vi "Main.vi"() -> ()   [LabVIEW 2016]
uses:
  type defs/action buttons.ctl
  type defs/mode buttons.ctl
  <vilib>/picture/picture.llb/imagedata.ctl
  type defs/state.ctl
  type defs/data.ctl
  <vilib>/vision/Image Controls.llb/IMAQ Image.ctl
  type defs/task.ctl
  <vilib>/vision/NI_Vision_Development_Module.lvlib
panel:
  in  "# máximo\nde iterações":i32
  out "image":u8[](array[numeric])
  out "image data":T1
  out "Array":T2(array[cluster])
  in  "K":u16
  in  "threshold (0 a 255)":u8
  out "Frame Rate":dbl
  in  "mode buttons":T3
  out "image display":T4(plugin-control)
  in  "action buttons":T5
  in  "Stop":bool
  # "Machine\nVision\nApp"
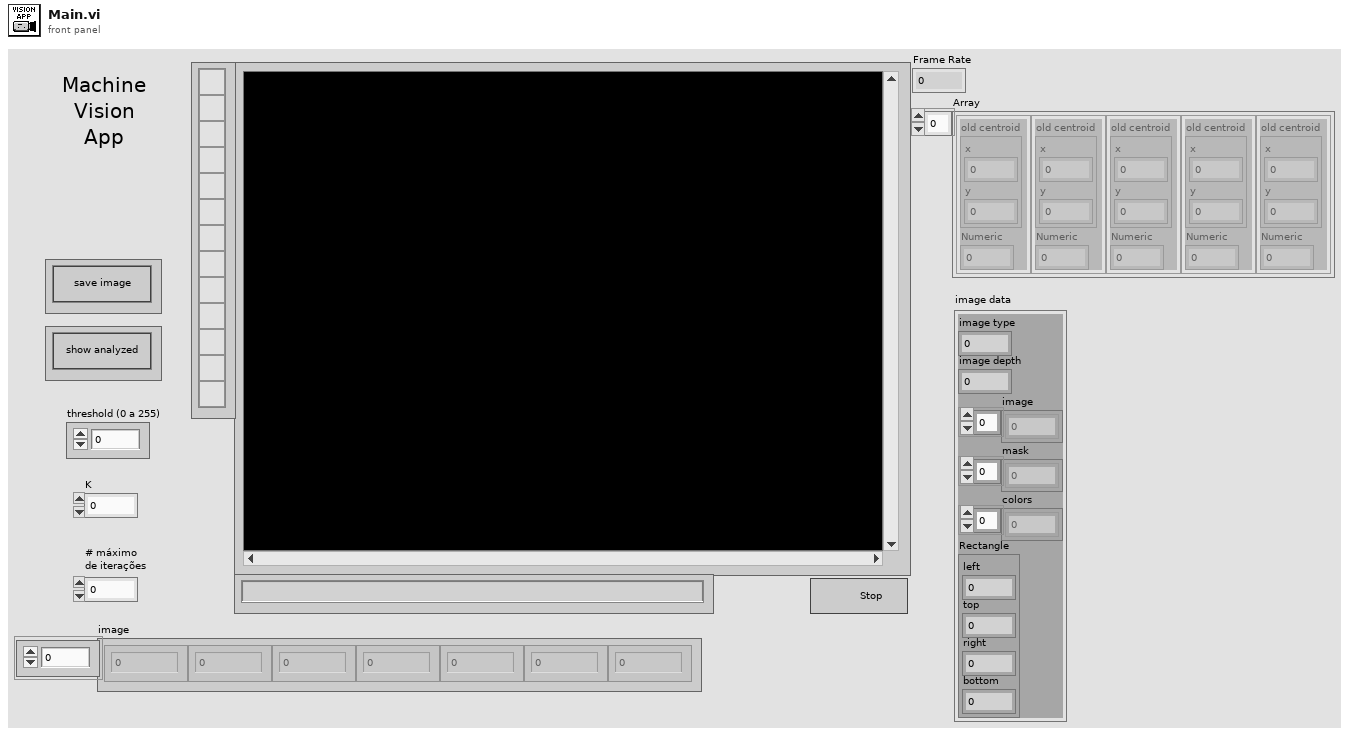
[diagram p1: front panel]
types:
  T1 = typedef "imagedata.ctl" = cluster{"image type":i32, "image depth":i32, "image":u8[], "mask":u8[], "colors":u32[], "Rectangle":cluster{"left":i16, "top":i16, "right":i16, "bottom":i16}}
  T2 = cluster{"old centroid":cluster{"x":dbl, "y":dbl}, "Numeric":i32}[]
  T3 = typedef "mode buttons.ctl" = cluster{"show analyzed":bool}
  T4 = typedef "IMAQ Image.ctl" = refnum<image>
  T5 = typedef "action buttons.ctl" = cluster{"save image":bool}
  T6 = typedef "data.ctl" = cluster{"save image":bool, "qsm":cluster{"Webcam image ref":T4, "Analyzed image ref":T4, "Stop webcam":bool}}
  T7 = typedef "state.ctl" = enum16{"(qsm) schedule", "(qsm) initialize", "(qsm) release", "(qsm) clean up", "(qsm) shutdown", "(myRIO) initialize", "(myRIO) clean up", "(myRIO) update ports", "(image) get", "(image) analyze", "(image) overlay", "(image) show", "save image", "state A", "state B", "state C", "state D", "state E", "state F", "state G", "state H"}
  T8 = cluster{"Desired Font (Application)":enum16{"User-specified Font", "Application Font", "System Font", "Dialog Font"}, "[User-specified Font]":cluster{"Font Name":string, "Size":i16, "Strikeout?":bool, "Italic?":bool, "Underline?":bool, "Outline?":bool, "Shadow?":bool, "Bold?":bool, "Rotation Angle":dbl}, "Horizontal Alignment":i16, "Vertical Alignment":i16}
  T9 = typedef "task.ctl" = T7[]
  T10 = typedef "Image Type" = u32
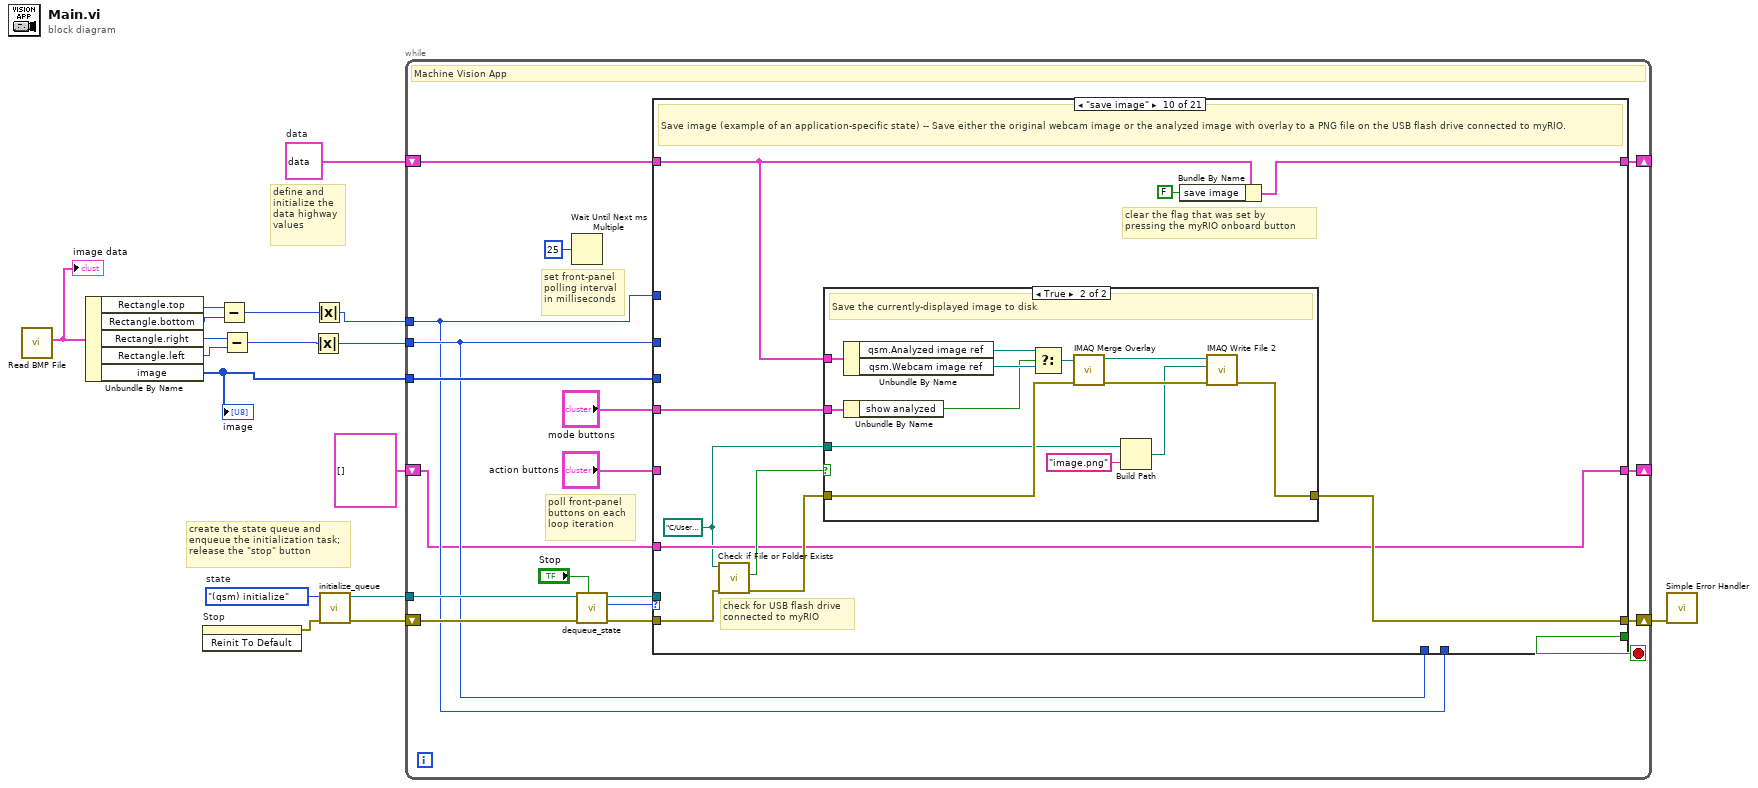
[diagram p0: block diagram]
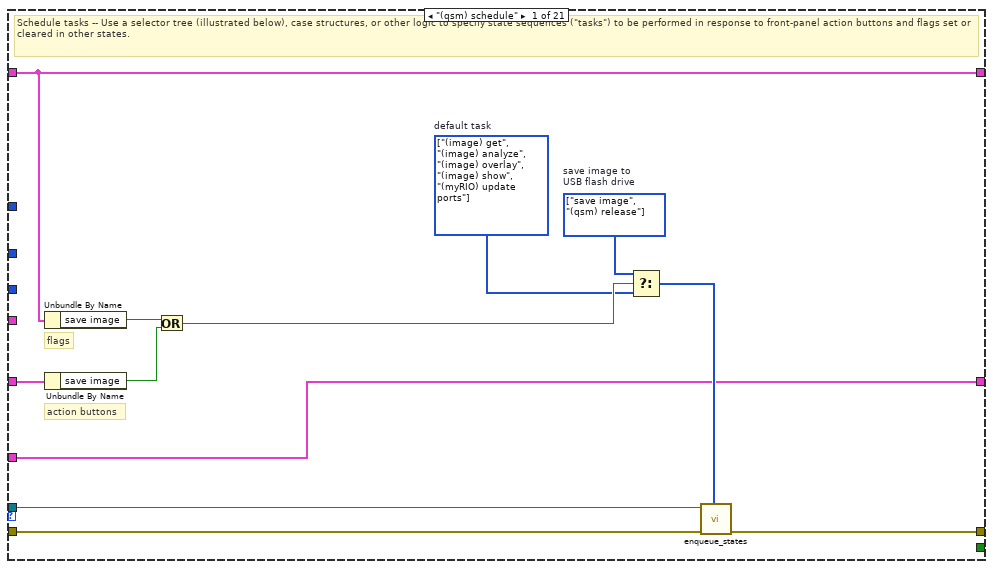
[diagram p2: hidden frame]
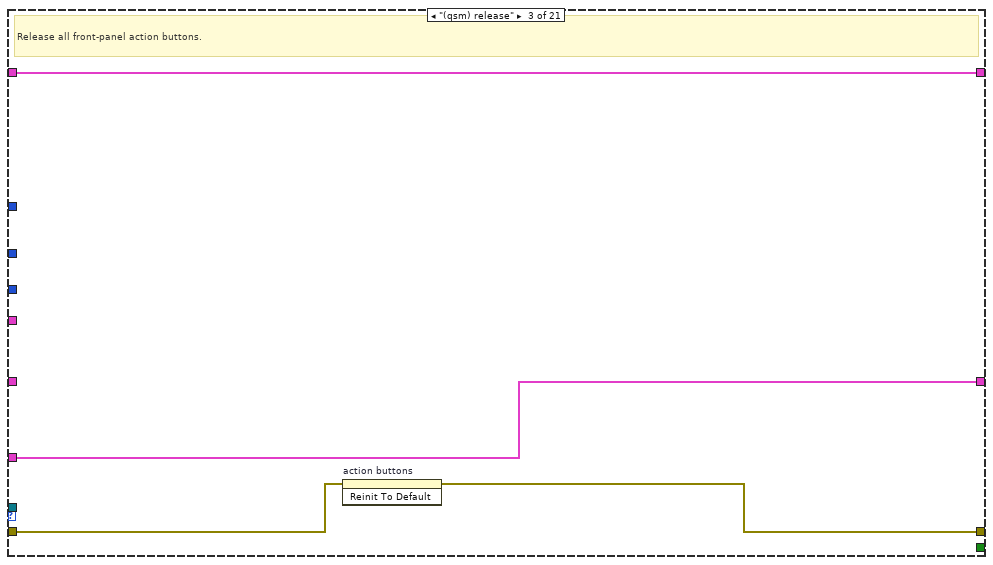
[diagram p4: hidden frame]
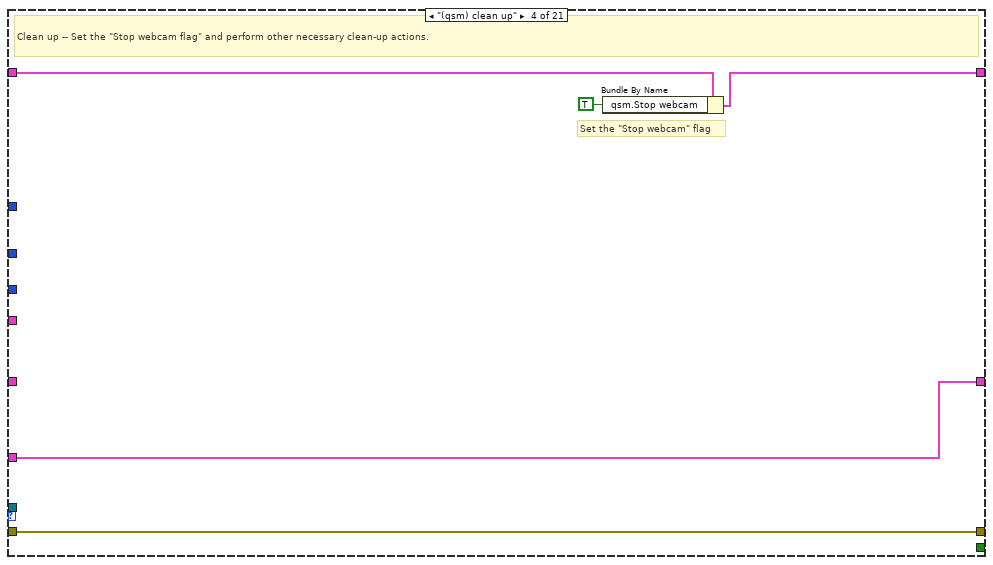
[diagram p5: hidden frame]
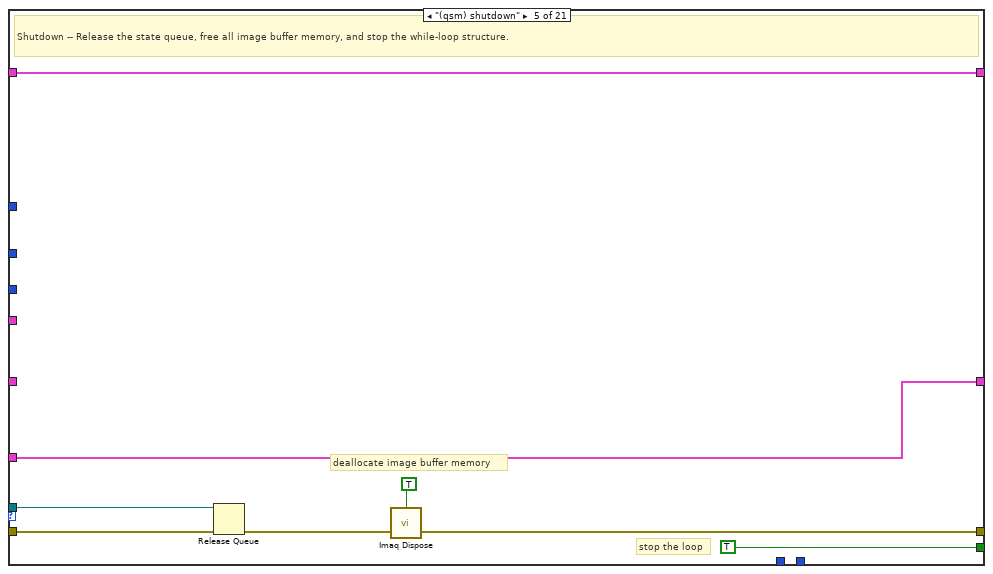
[diagram p6: hidden frame]
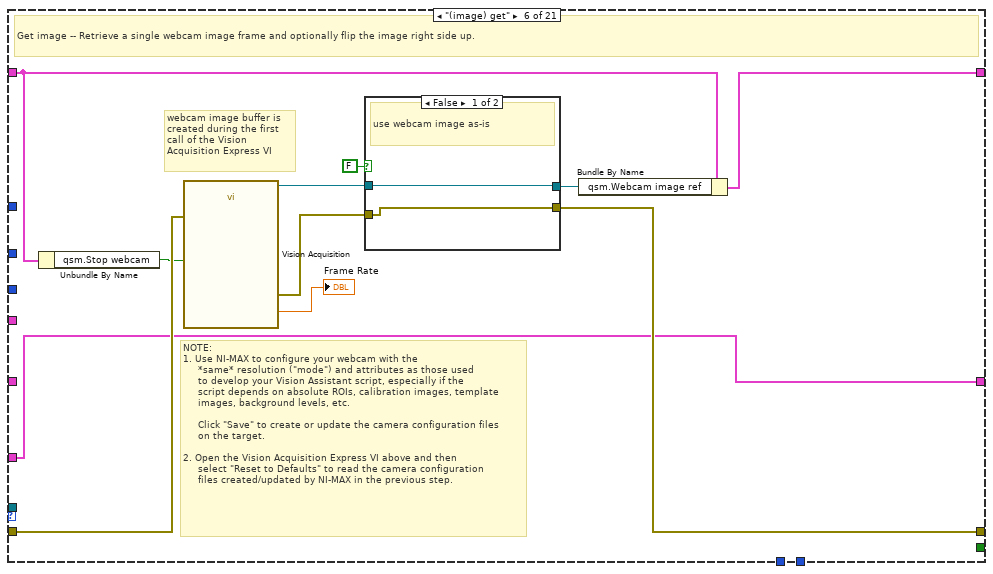
[diagram p7: hidden frame]
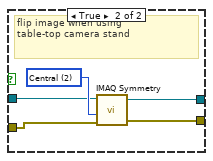
[diagram p8: hidden frame]
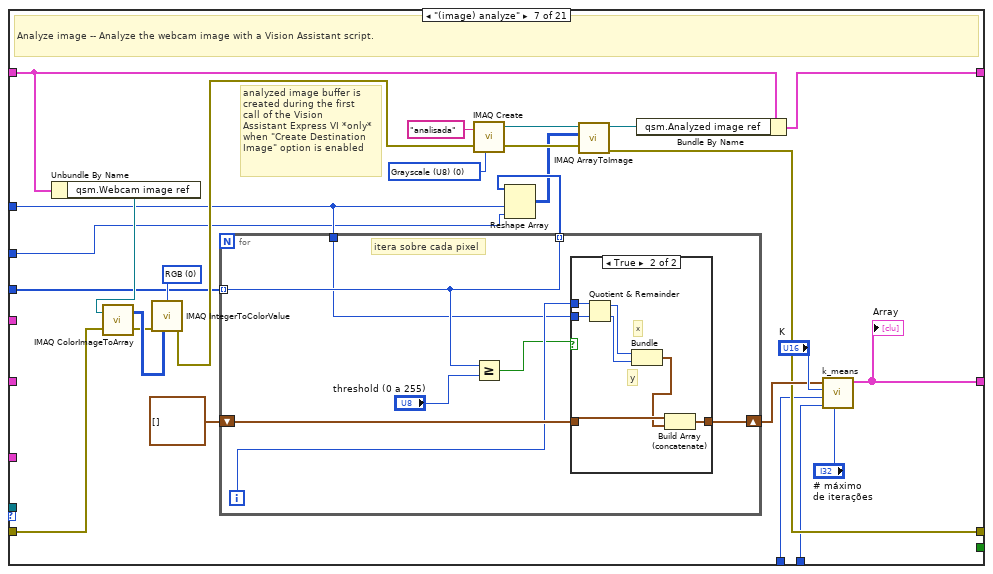
[diagram p9: hidden frame]
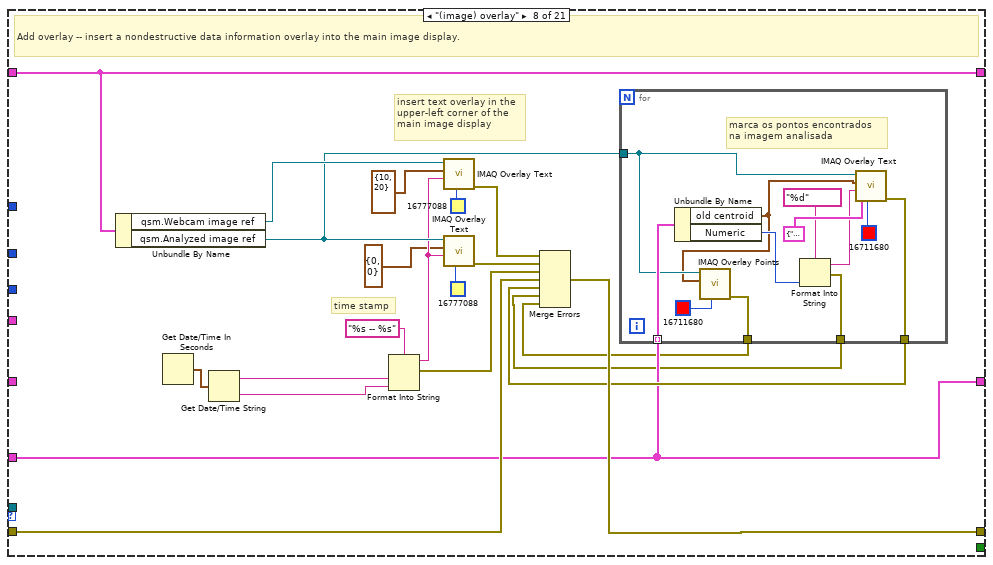
[diagram p11: hidden frame]
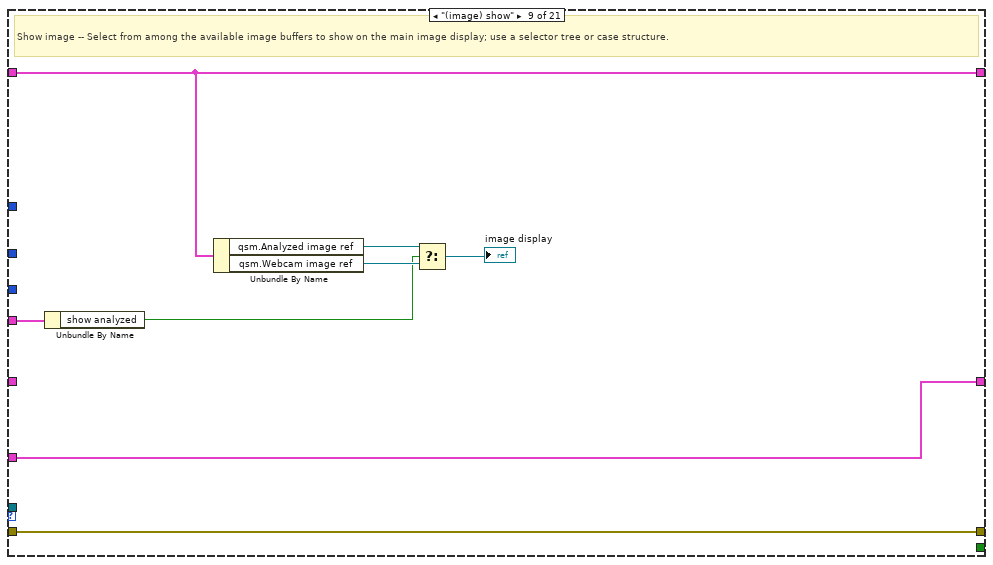
[diagram p12: hidden frame]
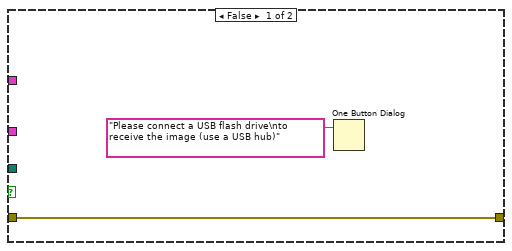
[diagram p13: hidden frame]
diagram:
  w16 = T6 {"save image"=FALSE, "qsm"={"Webcam image ref"=refnum, "Analyzed image ref"=refnum, "Stop webcam"=FALSE}}  # data
  w12 = state."(qsm) initialize"  # state
  # "define and \ninitialize the \ndata highway\nvalues"
  # "create the state queue and\nenqueue the initialization task;\nrelease the \"stop\" button"
  n1 = call <vilib>:"Read BMP File.vi"() -> ("image data"=w11:T1)  [unwired: 9 in, 2 out]
  "image data" <- w11
  n2 = Unbundle By Name(w11) -> ("Rectangle.top"=w7:i16, "Rectangle.bottom"=w6:i16, "Rectangle.right"=w9:i16, "Rectangle.left"=w8:i16, "image"=w10:u8[])
  "image" <- w10
  n3 = invoke on="Stop" class="Bool" method="Reinit To Default"() -> (error out=w13:errorcluster)  [unwired: 3 in, 2 out]
  n4 = Subtract(x=w7, y=w6) -> (x-y=w5:i16)
  n5 = Subtract(x=w9, y=w8) -> (x-y=w3:i16)
  n6 = Absolute Value(x=w3) -> (abs(x)=w2:i16)
  n7 = Absolute Value(x=w5) -> (abs(x)=w4:i16)
  n8 = call "initialize_queue.vi"("error in (no error)"=w13, "state"=w12) -> ("error out"=w15:errorcluster, "queue out"=w14:refnum<queue>)  [unwired: 8 in]
  n9 = while {
    shift-right: [w23] -> w17
    shift-left: w15 -> [w31]
    tunnel: w14 -> [w32]
    shift-right: [w25] -> _
    shift-left: w16 -> [w34]
    tunnel: w10 -> [w22]
    tunnel: w4 -> [w20]
    tunnel: w2 -> [w21]
    shift-right: [w19] -> _
    shift-left: T2 [] ("Array") -> [w18]
    stop <- w33 stop-if-true
    # "set front-panel\npolling interval\nin milliseconds"
    # "poll front-panel\nbuttons on each\nloop iteration"
    # "Machine Vision App"
    n10 = Wait Until Next ms Multiple(millisecond multiple=u32 25) -> ()  [unwired: 1 out]
    n11 = call "dequeue_state.vi"("stop"="Stop", "error in (no error)"=w31, "queue in"=w32) -> ("error out"=w24:errorcluster, "state"=w26:T7, "queue out"=w29:refnum<queue>)  [unwired: 6 in]
    n12 = case shown="\"save image\"" w26 {
      tunnel: w29 -> [w45 _ _ _ w65 _ _ _ _ _ _ _ _ _ _ _ _ _ _ _ _]
      tunnel: "action buttons" -> [w47 _ _ _ _ _ _ _ _ _ _ _ _ _ _ _ _ _ _ _ _]
      tunnel: w34 -> [w46 w50 w54 w58 w64 w72 w111 w136 w164 w177 w195 w198 w201 w204 w207 w210 w213 w216 w219 w222 w225]
      tunnel: [_ _ _ _ TRUE _ _ _ _ _ _ _ _ _ _ _ _ _ _ _ _] -> w33
      tunnel: "mode buttons" -> [_ _ _ _ _ _ _ _ w163 w173 _ _ _ _ _ _ _ _ _ _ _]
      tunnel: [w46 w50 w54 w57 w64 w77 w110 w136 w164 w176 w195 w198 w201 w204 w207 w210 w213 w216 w219 w222 w225] -> w25
      tunnel: w24 -> [w44 w49 w53 w56 w66 w78 w97 w135 w161 w174 w194 w197 w200 w203 w206 w209 w212 w215 w218 w221 w224]
      tunnel: [w37 w49 w52 w56 w61 w70 w96 w134 w161 w170 w194 w197 w200 w203 w206 w209 w212 w215 w218 w221 w224] -> w23
      tunnel: w22 -> [_ _ _ _ _ _ w95 _ _ _ _ _ _ _ _ _ _ _ _ _ _]
      tunnel: w20 -> [_ _ _ _ _ _ w90 _ _ _ _ _ _ _ _ _ _ _ _ _ _]
      tunnel: w21 -> [_ _ _ _ _ _ w89 _ _ _ _ _ _ _ _ _ _ _ _ _ _]
      tunnel: w21 -> [_ _ _ _ _ _ w88 _ _ _ _ _ _ _ _ _ _ _ _ _ _]
      tunnel: w20 -> [_ _ _ _ _ _ w87 _ _ _ _ _ _ _ _ _ _ _ _ _ _]
      tunnel: [w36 w48 w51 w55 w60 w68 w86 w131 w160 w169 w193 w196 w199 w202 w205 w208 w211 w214 w217 w220 w223] -> w19
      tunnel: w18 -> [w36 w48 w51 w55 w60 w68 _ w131 w160 w169 w193 w196 w199 w202 w205 w208 w211 w214 w217 w220 w223]
      frame "(qsm) schedule" {
        w40 = T9 [enum."save image", enum."(qsm) release"] items=["(qsm) schedule", "(qsm) initialize", "(qsm) release", "(qsm) clean up", "(qsm) shutdown", "(myRIO) initialize", "(myRIO) clean up", "(myRIO) update ports", "(image) get", "(image) analyze", "(image) overlay", "(image) show", "save image", "state A", "state B", "state C", "state D", "state E", "state F", "state G", "state H"]  # save image to USB flash drive
        w38 = T9 [enum."(image) get", enum."(image) analyze", enum."(image) overlay", enum."(image) show", enum."(myRIO) update ports"] items=["(qsm) schedule", "(qsm) initialize", "(qsm) release", "(qsm) clean up", "(qsm) shutdown", "(myRIO) initialize", "(myRIO) clean up", "(myRIO) update ports", "(image) get", "(image) analyze", "(image) overlay", "(image) show", "save image", "state A", "state B", "state C", "state D", "state E", "state F", "state G", "state H"]  # default task
        # "action buttons"
        # "flags"
        # "Schedule tasks -- Use a selector tree (illustrated below), case structures, or other logic to specify state sequences (\"tasks\") to be performed in response to front-panel action buttons and flags set or cleared in other states."
        n13 = Unbundle By Name "Unbundle By Name"(w46) -> ("save image"=w43:bool)
        n14 = Unbundle By Name(w47) -> ("save image"=w42:bool)
        n15 = Or(x=w43, y=w42) -> (x .or. y?=w41:bool)
        n16 = Select(t=w40, s=w41, f=w38) -> (s? t:f=w39:T9)
        n17 = call "enqueue_states.vi"("task"=w39, "error in"=w44, "queue in"=w45) -> ("error out"=w37:errorcluster)  [unwired: 7 in, 1 out]
      }
      frame "(qsm) initialize" {
        # "Initialize -- Allocate memory for additional image buffers, if necessary, and perform other one-time initialization steps."
      }
      frame "(qsm) release" {
        # "Release all front-panel action buttons."
        n18 = invoke on="action buttons" class="Clust (strict)" method="Reinit To Default"(error in=w53) -> (error out=w52:errorcluster)  [unwired: 2 in, 2 out]
      }
      frame "(qsm) clean up" {
        # "Set the \"Stop webcam\" flag"
        # "Clean up -- Set the \"Stop webcam flag\" and perform other necessary clean-up actions."
        n19 = Bundle By Name(cluster=w58, "qsm.Stop webcam"=TRUE) -> (w57:T6)
      }
      frame "(qsm) shutdown" {
        # "deallocate image buffer memory"
        # "stop the loop"
        # "Shutdown -- Release the state queue, free all image buffer memory, and stop the while-loop structure."
        n20 = Release Queue(queue=w65, error in (no error)=w66) -> (error out=w62:errorcluster)  [unwired: 1 in, 2 out]
        n21 = call "Imaq Dispose"("All Images? (No)"=TRUE, "error in (no error)"=w62) -> ("error out"=w61:errorcluster)  [unwired: 4 in]
      }
      frame "(image) get" {
        # "webcam image buffer is\ncreated during the first\ncall of the Vision\nAcquisition Express VI"
        # "NOTE:\n1. Use NI-MAX to configure your webcam with the\n     *same* resolution (\"mode\") and attributes as those used \n     to develop your Vision Assistant script, especially if the\n     script depends on absolute ROIs, calibration images, template\n     images, background levels, etc.\n \n     Click \"Save\" to create or update the camera configuration files\n     on the target.\n\n2. Open the Vision Acquisition Express VI above and then\n     select \"Reset to Defaults\" to read the camera configuration\n     files created/updated by NI-MAX in the previous step."
        # "Get image -- Retrieve a single webcam image frame and optionally flip the image right side up."
        n22 = Unbundle By Name(w72) -> ("qsm.Stop webcam"=w71:bool)
        n23 = call "Vision Acquisition"("Stop (F)"=w71, "error in"=w78) -> ("Image Out"=w76:T4, "Frame Rate"=→"Frame Rate":dbl, "error out"=w74:errorcluster)  [unwired: 22 in, 1 out]
        n24 = case shown="False" FALSE {
          tunnel: w76 -> [w80 w84]
          tunnel: [w80 w83] -> w75
          tunnel: w74 -> [w79 w82]
          tunnel: [w79 w81] -> w70
          frame False {
            # "use webcam image as-is"
          }
          frame True {
            w85 = u32 2 items=["Horizontal", "Vertical", "Central", "1st Diagonal", "2nd Diagonal"] ("Type of Symmetry")
            # "flip image when using\ntable-top camera stand"
            n25 = call "IMAQ Symmetry"("error in (no error)"=w82, "Type of Symmetry"=w85, "Image Src"=w84) -> ("error out"=w81:errorcluster, "Image Dst Out"=w83:T4)  [unwired: 2 in]
          }
        }
        n26 = Bundle By Name(cluster=w72, "qsm.Webcam image ref"=w75) -> (w77:T6)
      }
      frame "(image) analyze" {
        w105 = T10 0 items=["Grayscale (U8)", "Grayscale (I16)", "Grayscale (SGL)", "Complex (CSG)", "RGB (U32)", "HSL (U32)", "RGB (U64)", "Grayscale (U16)"] ("Image Type")
        w107 = u16 0 items=["RGB", "HSL", "HSV", "HSI"] ("Color Mode")
        # "analyzed image buffer is\ncreated during the first\ncall of the Vision\nAssistant Express VI *only*\nwhen \"Create Destination\nImage\" option is enabled"
        # "Analyze image -- Analyze the webcam image with a Vision Assistant script."
        n27 = Unbundle By Name "Unbundle By Name"(w111) -> ("qsm.Webcam image ref"=w103:T4)
        n28 = call "IMAQ ColorImageToArray"("Image"=w103, "error in (no error)"=w97) -> ("Image Pixels (U32)"=w109:u32[][], "error out"=w108:errorcluster)  [unwired: 2 in, 1 out]
        n29 = call "IMAQ IntegerToColorValue"("error in (no error)"=w108, "2D U32 array"=w109, "Color Mode"=w107) -> ("error out"=w101:errorcluster)  [unwired: 2 in, 3 out]
        n30 = for {
          tunnel: [w115] -> w93 mode=indexing
          shift-right: [w118] -> w99
          shift-left: cluster{dbl, dbl}[] [] -> [w117]
          tunnel: w95 -> [w115] mode=indexing
          tunnel: w90 -> [w112]
          i -> [w116]
          # "itera sobre cada pixel"
          n31 = Greater Or Equal?(x=w115, y="threshold (0 a 255)") -> (x >= y?=w113:bool)
          n32 = case shown="True" w113 {
            tunnel: [w119 w126] -> w118
            tunnel: w117 -> [w119 w125]
            tunnel: w116 -> [_ w124]
            tunnel: w112 -> [_ w123]
            frame False {
            }
            frame True {
              # "y"
              # "x"
              n33 = Quotient & Remainder(x=w124, y=w123) -> (x-y*floor(x/y)=w122:i32, floor(x/y)=w121:i32)
              n34 = Bundle(w122, w121) -> (w120:cluster{i32, i32})  [unwired: 1 in]
              n35 = Build Array (concatenate)(w125, w120) -> (w126:cluster{dbl, dbl}[])
            }
          }
        }
        n36 = call "IMAQ Create"("Image Name"="analisada", "Image Type"=w105, "error in (no error)"=w101) -> ("New Image"=w104:T4, "error out"=w102:errorcluster)  [unwired: 2 in]
        n37 = Reshape Array(w93, w90, w89) -> (w92:u8[][])
        n38 = call "IMAQ ArrayToImage"("error in (no error)"=w102, "Image Pixels (U8)"=w92, "Image"=w104) -> ("error out"=w96:errorcluster, "Image Out"=w91:T4)  [unwired: 7 in]
        n39 = Bundle By Name "Bundle By Name"(cluster=w111, "qsm.Analyzed image ref"=w91) -> (w110:T6)
        n40 = call "k_means.vi"("# máximo de iterações"="# máximo\nde iterações", "altura (pixels)"=w87, "largura (pixels)"=w88, "K"="K", "point array"=w99) -> ("Array"=w86:T2)  [unwired: 5 in, 1 out]
        "Array" <- w86
      }
      frame "(image) overlay" {
        # "time stamp"
        # "insert text overlay in the\nupper-left corner of the \nmain image display"
        # "Add overlay -- insert a nondestructive data information overlay into the main image display."
        n41 = Unbundle By Name "Unbundle By Name"(w136) -> ("qsm.Webcam image ref"=w145:T4, "qsm.Analyzed image ref"=w133:T4)
        n42 = Get Date/Time In Seconds() -> (seconds since 1Jan1904=w140:timestamp)
        n43 = Get Date/Time String(seconds (now)=w140) -> (date string=w139:string, time string=w138:string)  [unwired: 2 in]
        n44 = Format Into String "Format Into String"(format string="%s -- %s", w139, w138) -> (resulting string=w129:string, error out=w137:errorcluster)  [unwired: 2 in]
        n45 = call "IMAQ Overlay Text"("Text Color (black)"=u32 16777088, "String"=w129, "Origin"=cluster{"X":i32, "Y":i32} {"X"=10, "Y"=20}, "Image"=w145) -> ("error out"=w142:errorcluster)  [unwired: 6 in, 1 out]
        n46 = call "IMAQ Overlay Text"("Text Color (black)"=u32 16777088, "String"=w129, "Origin"=cluster{"X":i32, "Y":i32} {"X"=0, "Y"=0}, "Image"=w133) -> ("error out"=w143:errorcluster)  [unwired: 6 in, 1 out]
        n47 = for {
          tunnel: w133 -> [w151]
          tunnel: [w159] -> w132
          tunnel: w131 -> [w158] mode=indexing
          tunnel: [w152] -> w130
          tunnel: [w149] -> w127
          # "marca os pontos encontrados\nna imagem analisada"
          n48 = Unbundle By Name(w158) -> ("old centroid"=w150:cluster{"x":dbl, "y":dbl}, "Numeric"=w154:i32)
          n49 = call "IMAQ Overlay Points"("Color"=u32 16711680, "Point"=w150, "Image"=w151) -> ("error out"=w149:errorcluster)  [unwired: 7 in, 1 out]
          n50 = Format Into String(format string="%d", w154) -> (resulting string=w153:string, error out=w152:errorcluster)  [unwired: 2 in]
          n51 = call "IMAQ Overlay Text"("Text Color (black)"=u32 16711680, "Font, Size & Style"=T8 {"Desired Font (Application)"=enum."Application Font", "[User-specified Font]"={"Font Name"="", "Size"=32, "Strikeout?"=FALSE, "Italic?"=FALSE, "Underline?"=FALSE, "Outline?"=FALSE, "Shadow?"=FALSE, "Bold?"=TRUE, "Rotation Angle"=0.0}, "Horizontal Alignment"=0, "Vertical Alignment"=0}, "String"=w153, "Origin"=w150, "Image"=w151) -> ("error out"=w159:errorcluster)  [unwired: 5 in, 1 out]
        }
        n52 = Merge Errors "Merge Errors"(w142, w143, w137, w135, w132, w130, w127) -> (w134:errorcluster)
      }
      frame "(image) show" {
        # "Show image -- Select from among the available image buffers to show on the main image display; use a selector tree or case structure."
        n53 = Unbundle By Name "Unbundle By Name"(w163) -> ("show analyzed"=w162:bool)
        n54 = Unbundle By Name "Unbundle By Name"(w164) -> ("qsm.Analyzed image ref"=w167:T4, "qsm.Webcam image ref"=w166:T4)
        n55 = Select(t=w167, s=w162, f=w166) -> (s? t:f=→"image display":T4)
      }
      frame "save image" {
        w168 = path "C:/Users/renan/Desktop/PFC/NI_myRIO_Vision_Essentials_Guide/machine vision app/qsm" ("path")
        # "check for USB flash drive\nconnected to myRIO"
        # "clear the flag that was set by\npressing the myRIO onboard button"
        # "Save image (example of an application-specific state) -- Save either the original webcam image or the analyzed image with overlay to a PNG file on the USB flash drive connected to myRIO."
        n56 = call <vilib>:"Check if File or Folder Exists.vi"("error in (no error)"=w174, "path"=w168) -> ("error out"=w171:errorcluster, "file or folder exists?"=w172:bool)  [unwired: 7 in, 1 out]
        n57 = case shown="True" w172 {
          tunnel: w177 -> [_ w190]
          tunnel: w173 -> [_ w189]
          tunnel: [w178 w188] -> w170
          tunnel: w171 -> [w178 w186]
          tunnel: w168 -> [_ w182]
          frame False {
            n58 = One Button Dialog(message="Please connect a USB flash drive\nto receive the image (use a USB hub)") -> ()  [unwired: 1 in, 1 out]
          }
          frame True {
            # "Save the currently-displayed image to disk"
            n59 = Unbundle By Name(w190) -> ("qsm.Analyzed image ref"=w185:T4, "qsm.Webcam image ref"=w191:T4)
            n60 = Unbundle By Name(w189) -> ("show analyzed"=w187:bool)
            n61 = Select(t=w185, s=w187, f=w191) -> (s? t:f=w184:T4)
            n62 = call "IMAQ Merge Overlay"("error in (no error)"=w186, "Image Src"=w184) -> ("error out"=w192:errorcluster, "Image Dst Out"=w183:T4)  [unwired: 8 in]
            n63 = Build Path(base path=w182, name or relative path="image.png") -> (appended path=w181:path)
            n64 = call-poly "IMAQ Write File 2"("error in (no error)"=w192, "File Path"=w181, "Image"=w183) -> ("error out"=w188:errorcluster)  [unwired: 7 in, 1 out]
          }
        }
        n65 = Bundle By Name(cluster=w177, "save image"=FALSE) -> (w176:T6)
      }
      frame "state A" {
        # "Expansion State A"
      }
      frame "state B" {
        # "Expansion State B"
      }
      frame "state C" {
        # "Expansion State C"
      }
      frame "state D" {
        # "Expansion State D"
      }
      frame "state E" {
        # "Expansion State E"
      }
      frame "state F" {
        # "Expansion State F"
      }
      frame "state G" {
        # "Expansion State G"
      }
      frame "state H" {
        # "Expansion State H"
      }
      frame "(myRIO) initialize" {
      }
      frame "(myRIO) clean up" {
      }
      frame "(myRIO) update ports" {
      }
    }
  }
  n66 = call <vilib>:"Simple Error Handler.vi"("error in (no error)"=w17) -> ()  [unwired: 4 in, 5 out]
